vi "Write Channels Array.vi"(8 "error in (no error)":errorcluster, 10 "channel array":T1(array[cluster]), 11 "Y (N Ch) in":refnum<class "Y (N Ch).lvclass">) -> (0 "error out":errorcluster, 3 "Y (N Ch) out":refnum<class "Y (N Ch).lvclass">)   [LabVIEW 2017, in "Y (N Ch).lvclass"]
uses:
  <vilib>/addons/_NISVFA/_Shared subVIs/Data Objects/Y (DBL)/Y (N Ch).lvclass
  <vilib>/addons/_NISVFA/_Shared subVIs/Data Objects/Y (DBL)/Y (N Ch).lvclass/Y (N Ch).ctl
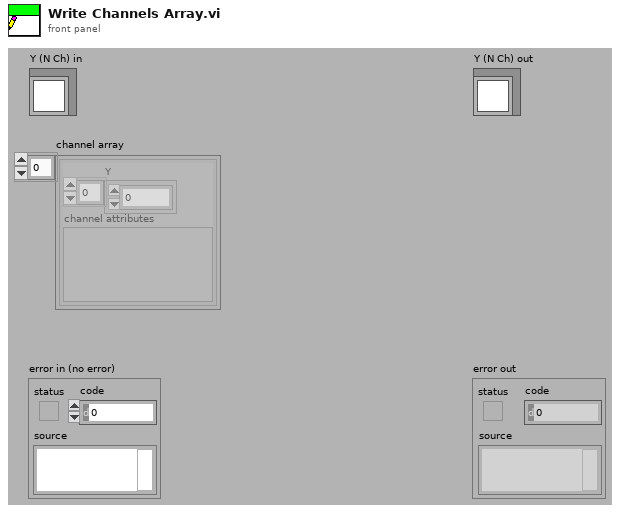
[diagram p1: front panel]
types:
  T1 = cluster{"Y":dbl[], "channel attributes":variant}[]
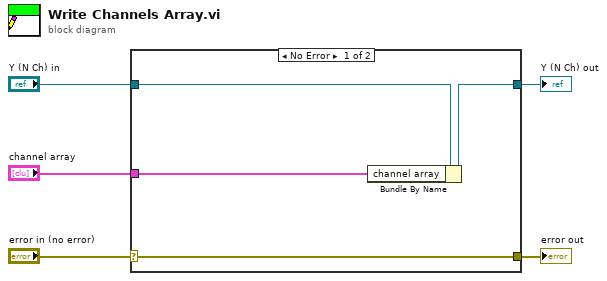
[diagram p0: block diagram]
diagram:
  n1 = case shown="No Error" "error in (no error)" {
    selector: "error in (no error)" -> [w9 w10]
    tunnel: [w9 w10] -> w4
    tunnel: [w7 w11] -> w2
    tunnel: "Y (N Ch) in" -> [w8 w11]
    tunnel: "channel array" -> [w6 _]
    frame No Error {
      n2 = Bundle By Name(cluster=w8, "channel array"=w6) -> (w7:refnum<class "Y (N Ch).lvclass">)
    }
    frame Error {
    }
  }
  "error out" <- w4
  "Y (N Ch) out" <- w2
